vi "Calibrate Volts.vi"(6 "Delay Time (s)":dbl=1.0, 8 "error in (no error)":errorcluster, 9 "COM Port":string="COM3", 10 "Device Name":string, 11 "Voltage":T1) -> (0 "error out":errorcluster, 1 "Report Text":string, 3 "Return Code":i32)   [LabVIEW 2015]
doc: "This vi will write to the DAQ to set the relays for the selected test and then set the calibrator and execute the spancalibration DLL"
uses:
  DAQ/Voltages.ctl
  DAQ/Relay Modes.ctl
  DAQ/Channels_v2.ctl
panel:
  # "`"
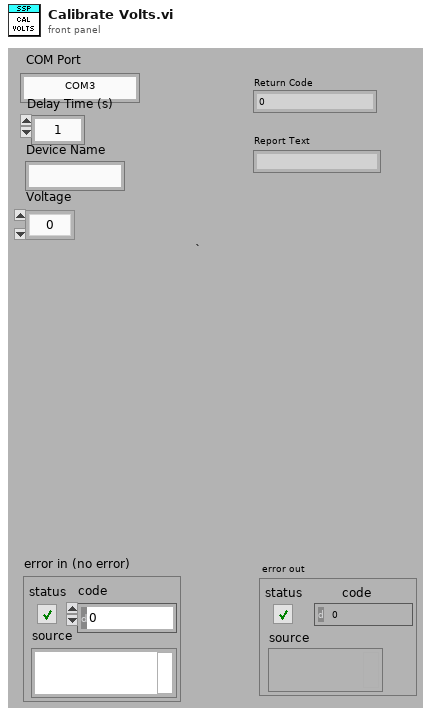
[diagram p1: front panel]
types:
  T1 = typedef "Voltages.ctl" = enum16{"0", "1", "2", "5", "10", "20", "50", "100", "200", "400"}
  T2 = typedef "Channels_v2.ctl" = enum16{"All Off", "Channel 4", "Channel 3", "4,3", "Channel 2", "4,2", "3,2", "4,3,2,", "Channel 1", "4,1", "3,1", "4,3,1", "2,1", "4,2,1", "3,2,1", "All On"}
  T3 = typedef "Relay Modes.ctl" = enum16{"All Off", "Short", "Ohms", "Fluke", "Daq AO 0"}
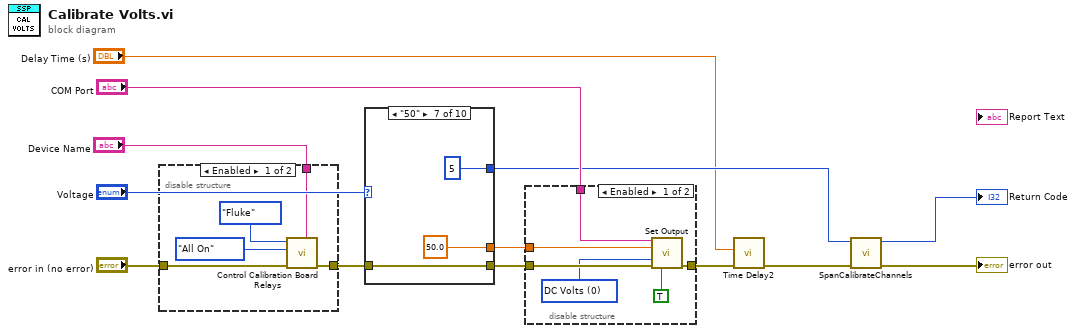
[diagram p0: block diagram]
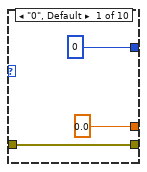
[diagram p4: hidden frame]
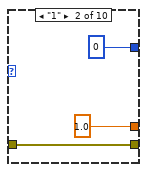
[diagram p5: hidden frame]
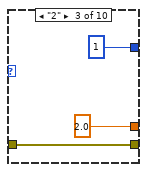
[diagram p6: hidden frame]
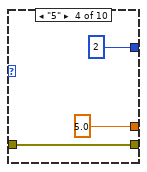
[diagram p7: hidden frame]
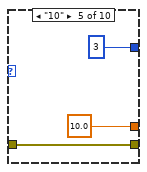
[diagram p8: hidden frame]
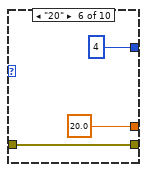
[diagram p9: hidden frame]
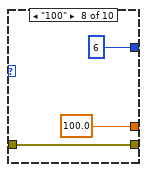
[diagram p10: hidden frame]
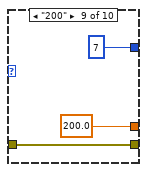
[diagram p11: hidden frame]
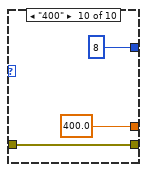
[diagram p12: hidden frame]
diagram:
  n1 = disable-structure shown="Enabled" {
    disable-tunnel: "error in (no error)" -> [w18 _]
    disable-tunnel: [w16 _] -> w11
    disable-tunnel: "Device Name" -> [w15 _]
    frame Enabled {
      n2 = call "Control Calibration Board Relays.vi"("Device Name"=w15, "error in"=w18, "Channels"=Channels_v2."All On", "Mode"=Relay_Modes."Fluke") -> ("error out"=w16:errorcluster)  [unwired: 7 in]
    }
    frame Disabled {
    }
  }
  n3 = case "Calibrate" shown="\"50\"" "Voltage" {
    tunnel: w11 -> [w21 w24 w27 w30 w33 w36 w39 w42 w45 w48]
    tunnel: [w21 w24 w27 w30 w33 w36 w39 w42 w45 w48] -> w10
    tunnel: [0.0 ("Primary Voltage") 1.0 ("Primary Voltage") 2.0 ("Primary Voltage") 5.0 ("Primary Voltage") 10.0 ("Primary Voltage") 20.0 ("Primary Voltage") 50.0 ("Primary Voltage") 100.0 ("Primary Voltage") 200.0 ("Primary Voltage") 400.0 ("Primary Voltage")] -> w8
    tunnel: [0 ("nScale") 0 ("nScale") 1 ("nScale") 2 ("nScale") 3 ("nScale") 4 ("nScale") 5 ("nScale") 6 ("nScale") 7 ("nScale") 8 ("nScale")] -> w5
    frame "0", Default {
    }
    frame "1" {
    }
    frame "2" {
    }
    frame "5" {
    }
    frame "10" {
    }
    frame "20" {
    }
    frame "50" {
    }
    frame "100" {
    }
    frame "200" {
    }
    frame "400" {
    }
  }
  n4 = disable-structure shown="Enabled" {
    disable-tunnel: w10 -> [w54 _]
    disable-tunnel: "COM Port" -> [w53 _]
    disable-tunnel: w8 -> [w51 _]
    disable-tunnel: [w50 _] -> w7
    frame Enabled {
      w52 = 0 items=["DC Volts", "AC Volts", "DC Current", "AC Current", "DC Power", "AC Power", "Dual DC Volts", "Dual AC Volts", "Resistance"] ("Output Type")
      n5 = call "Set Output.vi"("COM Port"=w53, "Primary Voltage"=w51, "Output Type"=w52, "error in"=w54, "Output Enabled"=TRUE) -> ("error out"=w50:errorcluster)  [unwired: 10 in]
    }
    frame Disabled {
    }
  }
  n6 = call "Time Delay2"("error in (no error)"=w7, "Delay Time (s)"="Delay Time (s)") -> ("error out"=w3:errorcluster)  [unwired: 9 in]
  n7 = call "SpanCalibrateChannels.vi"("error in"=w3, "nScale"=w5) -> ("error out"=→"error out":errorcluster, "Return Code"=→"Return Code":i32)  [unwired: 8 in]
